vi "SpinnyConfigCameraTrigger.vi"(8 "error in":errorcluster, 9 "Stepper #":u8=1, 10 "triggerInterval":u16, 11 "Arduino Resource":T1={"VISA resource"="", "Board Type"=enum."Uno", "Connection Type"=enum."USB / Serial", "Bytes Per Packet (15)"=15}) -> (0 "error out":errorcluster, 3 "Arduino Resource Out":T1={"VISA resource"="", "Board Type"=enum."Uno", "Connection Type"=enum."USB / Serial", "Bytes Per Packet (15)"=15})   [LabVIEW 2014]
doc: "set the interval (in steps of the indicated stepper) for a pulse to be sent to the indicated pin."
uses:
  <vilib>/LabVIEW Interface for Arduino/Type Defs/Arduino Resource.ctl
  <vilib>/LabVIEW Interface for Arduino/Type Defs/Board Type.ctl
  <vilib>/LabVIEW Interface for Arduino/LabVIEW Interface for Arduino.lvlib
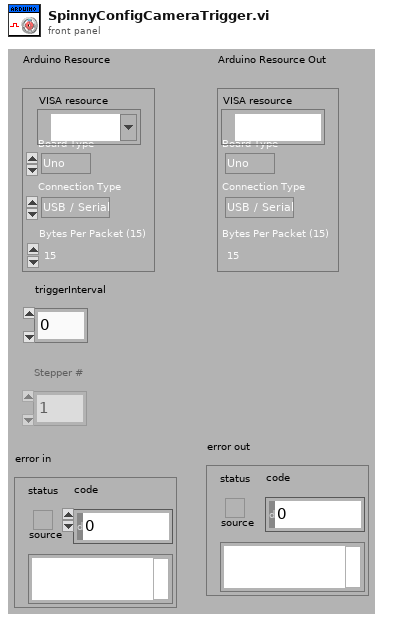
[diagram p1: front panel]
types:
  T1 = typedef "LabVIEW Interface for Arduino.lvlib/Arduino Resource.ctl" = cluster{"VISA resource":refnum<visa-resource-name>, "Board Type":T2, "Connection Type":enum8{"USB / Serial"}, "Bytes Per Packet (15)":u8}
  T2 = typedef "LabVIEW Interface for Arduino.lvlib/Board Type.ctl" = enum16{"Uno", "Dimuelanove w/Atmega 328", "Mega 2560"}
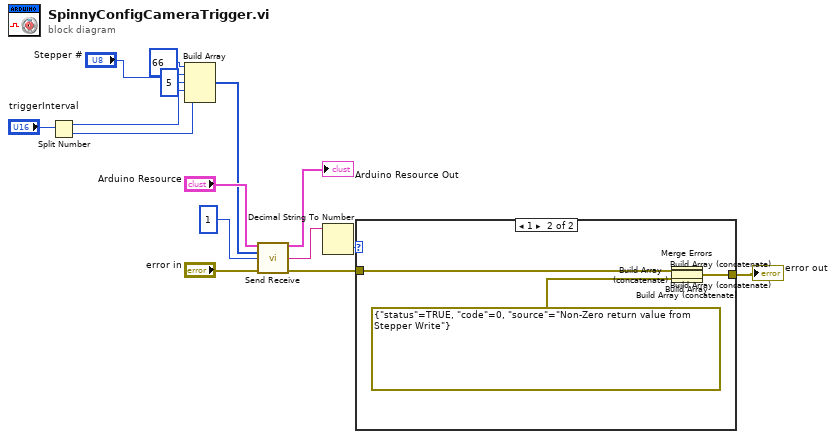
[diagram p0: block diagram]
diagram:
  n1 = Split Number(x="triggerInterval") -> (hi(x)=w2:u8, lo(x)=w1:u8)
  n2 = Build Array(u8 66, "Stepper #", u8 5 ("element"), w2, w1) -> (w12:u8[])
  n3 = call <vilib>:"Send Receive.vi"("Arduino Resource"="Arduino Resource", "Data"=w12, "Bytes To Read (0)"=u8 1, "error in"="error in") -> ("Arduino Resource"=→"Arduino Resource Out":T1, "Read Buffer"=w6:string, "error out"=w7:errorcluster)  [unwired: 9 in]
  n4 = Decimal String To Number(string=w6) -> (number=w9:i32)  [unwired: 2 in, 1 out]
  n5 = case shown="1" w9 {
    tunnel: w7 -> [w16 w24]
    tunnel: [w16 w23] -> w8
    frame 0, Default {
    }
    frame 1 {
      n6 = Build Array(w24, errorcluster {"status"=TRUE, "code"=0, "source"="Non-Zero return value from Stepper Write"} ("error in")) -> (w21:errorcluster[])
      n7 = Build Array (concatenate)(w21) -> (w20:errorcluster[])
      n8 = Build Array (concatenate)(w20) -> (w19:errorcluster[])
      n9 = Build Array (concatenate)(w19) -> (w18:errorcluster[])
      n10 = Build Array (concatenate)(w18) -> (w17:errorcluster[])
      n11 = Merge Errors(w17) -> (w23:errorcluster)
    }
  }
  "error out" <- w8
